vi "Initiate TS.vi"(8 "error in":errorcluster, 11 "DeepU Test Stand in":refnum<class "DeepU Test Stand.lvclass">) -> (0 "error out":errorcluster, 3 "DeepU Test Stand out":refnum<class "DeepU Test Stand.lvclass">)   [LabVIEW 2019, in "Test Stands.lvlib" / "DeepU Test Stand.lvclass"]
uses:
  DeepU Test Stand.lvclass
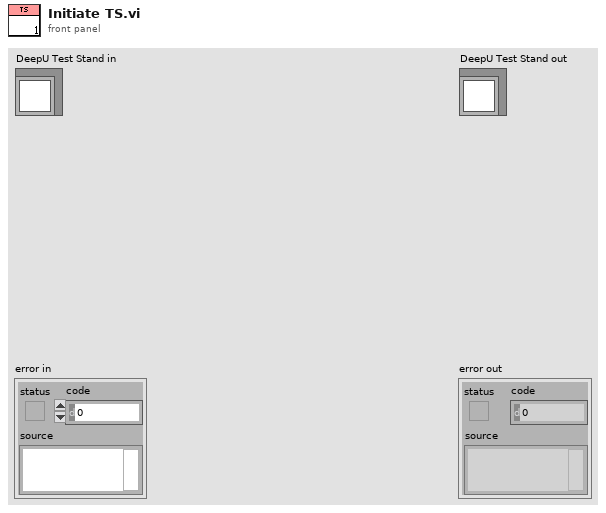
[diagram p1: front panel]
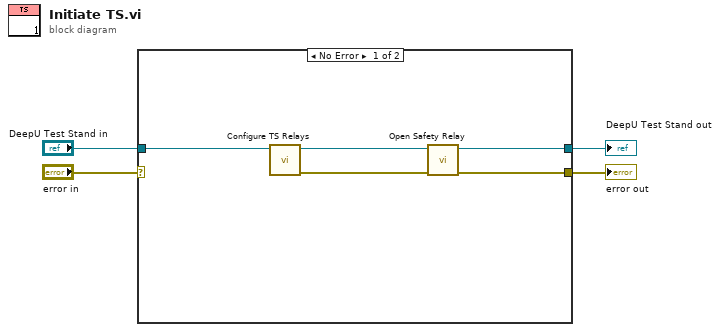
[diagram p0: block diagram]
diagram:
  n1 = case shown="No Error" "error in" {
    selector: "error in" -> [_ w11]
    tunnel: [w7 w11] -> w4
    tunnel: [w8 w10] -> w3
    tunnel: "DeepU Test Stand in" -> [w9 w10]
    frame No Error {
      n2 = call "Configure TS Relays.vi"("DeepU Test Stand in"=w9) -> ("error out"=w5:errorcluster, "DeepU Test Stand out"=w6:refnum<class "DeepU Test Stand.lvclass">)  [unwired: 9 in]
      n3 = call "Open Safety Relay.vi"("error in (no error)"=w5, "DeepU Test Stand in"=w6) -> ("error out"=w7:errorcluster, "DeepU Test Stand out"=w8:refnum<class "DeepU Test Stand.lvclass">)  [unwired: 8 in]
    }
    frame Error {
    }
  }
  "error out" <- w4
  "DeepU Test Stand out" <- w3
